vi "Find Variable Indices in Formula.vi"(8 "Error In":errorcluster, 9 "Variable":string, 11 "Formula String":string) -> (0 "Error Out":errorcluster, 1 "Array of Variable Indices":i32[](array[numeric]), 3 "Formula String (dup)":string)   [LabVIEW 2021, in "Formula.lvlib"]
uses:
  <userlib>/_OpenG.lib/array/array.llb/Remove Duplicates from 1D Array (I32)__ogtk.vi
  Formula.lvlib
  <userlib>/_OpenG.lib/array/array.llb/openg_array.lvlib
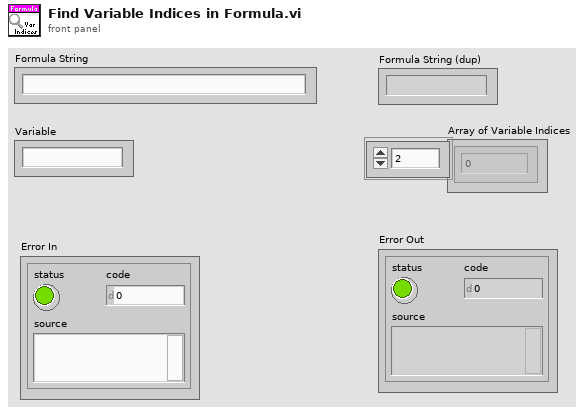
[diagram p1: front panel]
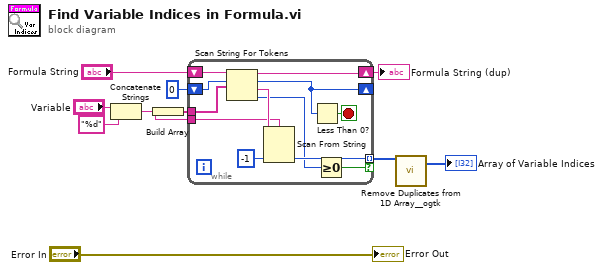
[diagram p0: block diagram]
diagram:
  n1 = Concatenate Strings("Variable", "%d" ("string")) -> (w6:string)
  n2 = Build Array(w6) -> (w10:string[])
  n3 = while {
    shift-right: [w21] -> w3
    shift-left: "Formula String" -> [w22]
    shift-right: [w19] -> _
    shift-left: 0 ("offset past token") -> [w20]
    tunnel: w10 -> [w16]
    tunnel: w6 -> [w15]
    tunnel: [w13] -> w4 mode=indexing if=w11
    stop <- w18 stop-if-true
    n4 = Scan String For Tokens(7:w16, 8:w20, 9:w22) -> (0:w12:i32, 1:w17:string, 2:w19:i32, 3:w21:string)  [unwired: 3 in]
    n5 = Scan From String(format string=w15, input string=w17, default 1=-1 ("default value 1")) -> (output 1=w13:i32)  [unwired: 2 in, 3 out]
    n6 = Less Than 0?(x=w19) -> (x < 0?=w18:bool)
    n7 = Greater Or Equal To 0?(x=w12) -> (x >= 0?=w11:bool)
  }
  "Formula String (dup)" <- w3
  n8 = call-poly <userlib>:"Remove Duplicates from 1D Array__ogtk.vi"("Input Array"=w4) -> ("Output Array"=→"Array of Variable Indices":i32[])  [unwired: 1 out]
  "Error Out" <- "Error In"
